vi "MGI Replace Cluster Element.vi"(8 "Error In":errorcluster, 9 "Data":variant, 10 "Name":string, 11 "Cluster In":variant) -> (0 "Error Out":errorcluster, 1 "Replaced?":bool, 3 "Cluster Out":variant)   [LabVIEW 2016]
doc: "This VI searches for an element or subelement in <b>Cluster In</b> named <b>Name</b> and replaces it with <b>Data</b>. If <b>Data</b> is the wrong size or if an element with <b>Name</b> cannot be found, then <b>Cluster In</b> will be returned for <b>Cluster Out</b>.\n\nAuthored by Robert C. Mortensen\nsupport@mooregoodideas.com\nwww.mooregoodideas.com\n\nCopyright (c) 2010, Moore Good Ideas, Inc.\n\nAll rights reserved.\n\nRedistribution and use in source and binary forms, with or without modification, are permitted provided that the following conditions are met:\n\n * Redistributions of source code must retain the above copyright notice, this list of conditions and the following disclaimer.\n * Redistributions in binary form must reproduce the above copyright notice, this list of conditions and the following disclaimer in the documentation and/or other materials provided with the distribution.\n * Neither the name of Moore Good Ideas, Inc. nor the names of its contributors may be used to endorse or promote products derived from this software without specific prior written permission.\n\nTHIS SOFTWARE IS PROVIDED BY THE COPYRIGHT HOLDERS AND CONTRIBUTORS \"AS IS\" AND ANY EXPRESS OR IMPLIED WARRANTIES, INCLUDING, BUT NOT LIMITED TO, THE IMPLIED WARRANTIES OF MERCHANTABILITY AND FITNESS FOR A PARTICULAR PURPOSE ARE DISCLAIMED. IN NO EVENT SHALL THE COPYRIGHT OWNER OR CONTRIBUTORS BE LIABLE FOR ANY DIRECT, INDIRECT, INCIDENTAL, SPECIAL, EXEMPLARY, OR CONSEQUENTIAL DAMAGES (INCLUDING, BUT NOT LIMITED TO, PROCUREMENT OF SUBSTITUTE GOODS OR SERVICES; LOSS OF USE, DATA, OR PROFITS; OR BUSINESS INTERRUPTION) HOWEVER CAUSED AND ON ANY THEORY OF LIABILITY, WHETHER IN CONTRACT, STRICT LIABILITY, OR TORT (INCLUDING NEGLIGENCE OR OTHERWISE) ARISING IN ANY WAY OUT OF THE USE OF THIS SOFTWARE, EVEN IF ADVISED OF THE POSSIBILITY OF SUCH DAMAGE."
uses:
  <vilib>/Utility/VariantDataType/VariantType.lvlib
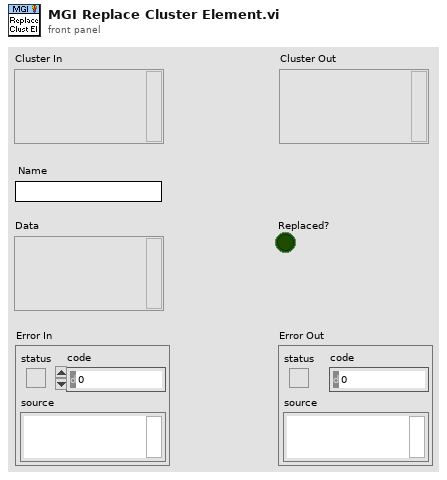
[diagram p1: front panel]
types:
  T1 = typedef "VariantType.lvlib/Type.ctl" = enum8{"Invalid Type", "Void", "I8", "I16", "I32", "I64", "U8", "U16", "U32", "U64", "Single Float", "Double Float", "Extended Float", "Single Complex", "Double Complex", "Extended Complex", "Enum U8", "Enum U16", "Enum U32", "Enum U64", "Single Float With Unit", "Double Float With Unit", "Extended Float With Unit", "Single Complex with Unit", "Double Complex with Unit", "Extended Complex with Unit", "Boolean", "String", "Path", "Picture", "Tag", "Array", "Cluster", "Variant", "LV Variant", "Waveform", "Timestamp", "Digital Waveform", "Digital Data", "ExpressData", "Refnum", "External Data", "VI", "Poly VI", "LabVIEW Class Instance", "Fixed Point"}
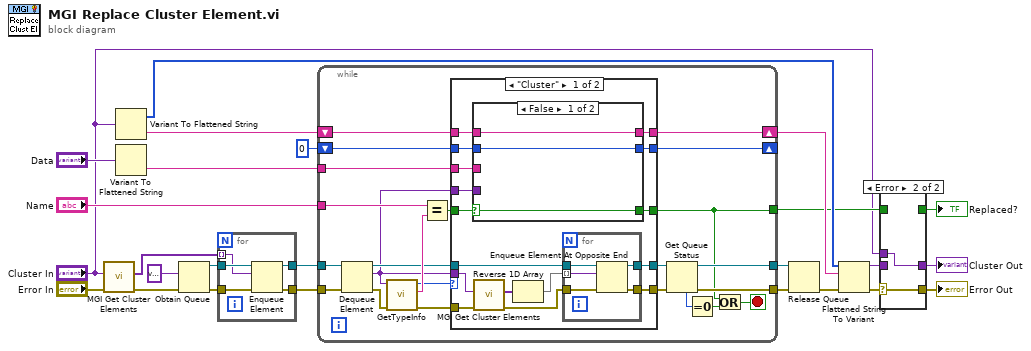
[diagram p0: block diagram]
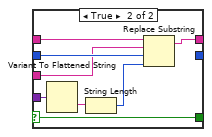
[diagram p3: hidden frame]
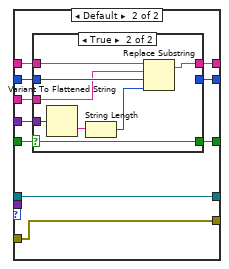
[diagram p4: hidden frame]
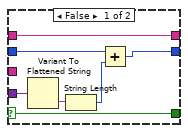
[diagram p5: hidden frame]
diagram:
  n1 = call <userlib>:"MGI Get Cluster Elements.vi"("Error In"="Error In", "Cluster"="Cluster In") -> ("Error Out"=w24:errorcluster, "Cluster Elements"=w21:variant[])  [unwired: 8 in]
  n2 = Variant To Flattened String(Variant="Cluster In") -> (data string=w17:string, 1:w8:i16[])
  n3 = Variant To Flattened String(Variant="Data") -> (data string=w13:string)  [unwired: 1 out]
  n4 = Obtain Queue(element data type=variant, error in (no error)=w24) -> (queue out=w22:refnum<queue>, error out=w23:errorcluster)  [unwired: 3 in, 1 out]
  n5 = for {
    tunnel: w23 -> [w30]
    tunnel: w22 -> [w29]
    tunnel: w21 -> [w28] mode=indexing
    tunnel: [w27] -> w18
    tunnel: [w26] -> w19
    n6 = Enqueue Element(queue=w29, element=w28, error in (no error)=w30) -> (queue out=w26:refnum<queue>, error out=w27:errorcluster)  [unwired: 1 in, 1 out]
  }
  n7 = while {
    tunnel: w19 -> [w52]
    tunnel: w18 -> [w53]
    shift-right: [w36] -> w12
    shift-left: w17 -> [w37]
    tunnel: "Name" -> [w46]
    shift-right: [w34] -> _
    shift-left: 0 ("length") -> [w38]
    tunnel: w13 -> [w35]
    tunnel: [w33] -> w11
    tunnel: [w32] -> w10
    tunnel: [w31] -> w2
    stop <- w49 stop-if-true
    n8 = Dequeue Element(queue=w52, error in (no error)=w53) -> (queue out=w44:refnum<queue>, element=w39:variant, error out=w48:errorcluster)  [unwired: 1 in, 1 out]
    n9 = call <vilib>:"GetTypeInfo.vi"("error in (no error)"=w48, "Variant"=w39) -> ("error out"=w43:errorcluster, "Name"=w47:string, "Type Enum"=w45:T1)  [unwired: 5 in, 2 out]
    n10 = Equal?(x=w46, y=w47) -> (x = y?=w40:bool)
    n11 = case shown="\"Cluster\"" w45 {
      tunnel: w44 -> [w63 w95]
      tunnel: w43 -> [w68 w94]
      tunnel: w39 -> [w69 _]
      tunnel: [w66 w94] -> w42
      tunnel: [w65 w95] -> w41
      tunnel: w40 -> [w61 w93]
      tunnel: w39 -> [w60 w88]
      tunnel: [w59 w92] -> w31
      tunnel: w38 -> [w58 w90]
      tunnel: w37 -> [w57 w89]
      tunnel: [w56 w87] -> w36
      tunnel: w35 -> [w55 w86]
      tunnel: [w54 w91] -> w34
      frame "Cluster" {
        n12 = case shown="False" w61 {
          selector: w61 -> [w72 w80]
          tunnel: [w72 w80] -> w59
          tunnel: w60 -> [_ w79]
          tunnel: w58 -> [w70 w76]
          tunnel: w57 -> [w71 w78]
          tunnel: [w71 w77] -> w56
          tunnel: w55 -> [_ w73]
          tunnel: [w70 _] -> w54
          frame False {
          }
          frame True {
            n13 = Variant To Flattened String(Variant=w79) -> (data string=w75:string)  [unwired: 1 out]
            n14 = String Length(string=w75) -> (length=w74:i32)
            n15 = Replace Substring(2:w74, 3:w76, 4:w73, 5:w78) -> (1:w77:string)  [unwired: 1 out]
          }
        }
        n16 = call <userlib>:"MGI Get Cluster Elements.vi"("Error In"=w68, "Cluster"=w69) -> ("Error Out"=w64:errorcluster, "Cluster Elements"=w67:variant[])  [unwired: 8 in]
        n17 = Reverse 1D Array(array=w67) -> (reversed array=w62:variant[])
        n18 = for {
          tunnel: w64 -> [w85]
          tunnel: w63 -> [w84]
          tunnel: w62 -> [w83] mode=indexing
          tunnel: [w82] -> w66
          tunnel: [w81] -> w65
          n19 = Enqueue Element At Opposite End(queue=w84, element=w83, error in (no error)=w85) -> (queue out=w81:refnum<queue>, error out=w82:errorcluster)  [unwired: 1 in, 1 out]
        }
      }
      frame Default {
        n20 = case shown="True" w93 {
          selector: w93 -> [w102 w110]
          tunnel: [w102 w110] -> w92
          tunnel: w88 -> [w100 w109]
          tunnel: w90 -> [w99 w106]
          tunnel: w89 -> [w101 w108]
          tunnel: [w101 w107] -> w87
          tunnel: w86 -> [_ w103]
          tunnel: [w96 _] -> w91
          frame False {
            n21 = Variant To Flattened String(Variant=w100) -> (data string=w98:string)  [unwired: 1 out]
            n22 = String Length(string=w98) -> (length=w97:i32)
            n23 = Add(x=w99, y=w97) -> (x+y=w96:i32)
          }
          frame True {
            n24 = Variant To Flattened String(Variant=w109) -> (data string=w105:string)  [unwired: 1 out]
            n25 = String Length(string=w105) -> (length=w104:i32)
            n26 = Replace Substring(2:w104, 3:w106, 4:w103, 5:w108) -> (1:w107:string)  [unwired: 1 out]
          }
        }
      }
    }
    n27 = Get Queue Status(queue=w41, error in (no error)=w42) -> (queue out=w32:refnum<queue>, error out=w33:errorcluster, # elements in queue=w51:i32)  [unwired: 1 in, 5 out]
    n28 = Equal To 0?(x=w51) -> (x = 0?=w50:bool)
    n29 = Or(x=w31, y=w50) -> (x .or. y?=w49:bool)
  }
  n30 = Release Queue(queue=w10, error in (no error)=w11) -> (error out=w9:errorcluster)  [unwired: 1 in, 2 out]
  n31 = Flattened String To Variant(4:w9, 6:w12, 7:w8) -> (0:w7:errorcluster, 3:w4:variant)
  n32 = case shown="Error" w7 {
    selector: w7 -> [w113 w114]
    tunnel: [w113 w114] -> w6
    tunnel: [w112 w115] -> w5
    tunnel: w4 -> [w112 _]
    tunnel: [w111 _] -> w3
    tunnel: w2 -> [w111 _]
    tunnel: "Cluster In" -> [_ w115]
    frame No Error {
    }
    frame Error {
    }
  }
  "Cluster Out" <- w5
  "Error Out" <- w6
  "Replaced?" <- w3
